vi "Measurement Data Convert (Harmonics).vi"(7 "Number of Harmonics Order (1)":i32=1 min=1 max=32, 8 "error in (no error)":errorcluster, 9 "Item Number Offset (1)":i32=1 min=1 max=32, 10 "Measurement Data (Empty)":string, 11 "VISA resource name":refnum<visa-resource-name>) -> (0 "error out":errorcluster, 1 "Measurement":dbl[][](array[numeric]), 2 "Function":string[](array[string]), 3 "VISA resource name out":refnum<visa-resource-name>)   [LabVIEW 2023, in "Yokogawa WT300 Series.lvlib"]
doc: "Transforms measurement datas into harmonics numeric data list values."
uses:
  Yokogawa WT300 Series.lvlib
panel:
  # "Total        DC            1             2              3             4"
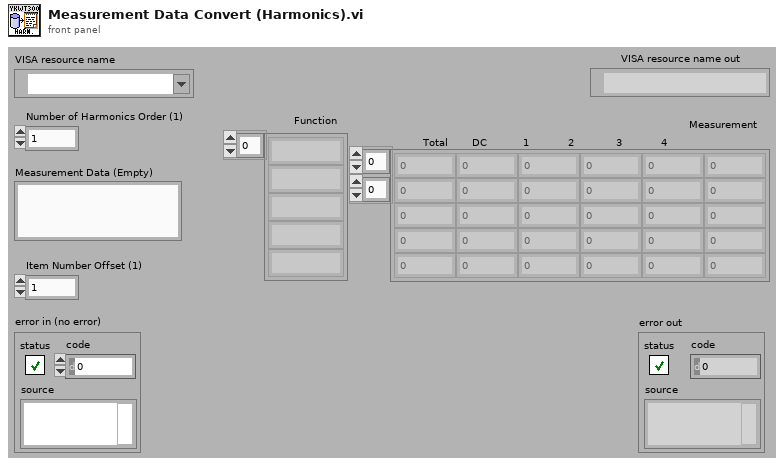
[diagram p1: front panel]
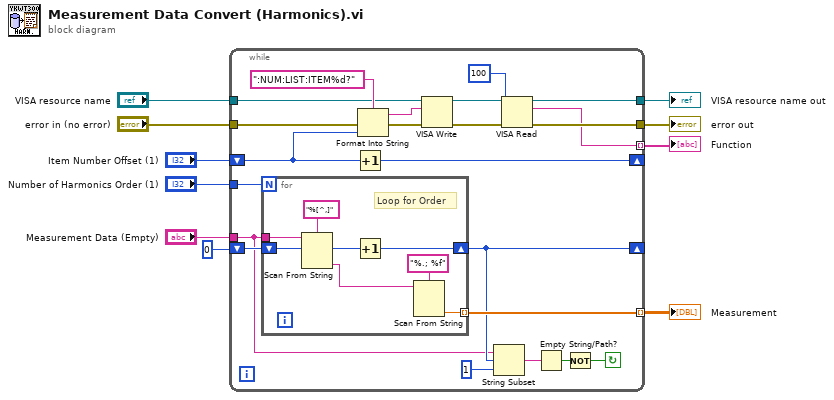
[diagram p0: block diagram]
diagram:
  n1 = while {
    tunnel: [w31] -> w4 mode=indexing
    tunnel: "Measurement Data (Empty)" -> [w23]
    shift-right: [w24] -> _
    shift-left: 0 -> [w32]
    tunnel: "VISA resource name" -> [w20]
    tunnel: "error in (no error)" -> [w22]
    shift-right: [w30] -> _
    shift-left: "Item Number Offset (1)" -> [w17]
    tunnel: [w13] -> w7
    tunnel: [w12] -> w6
    tunnel: [w11] -> w5 mode=indexing
    tunnel: "Number of Harmonics Order (1)" -> [w29]
    stop <- w25 continue-if-true
    n2 = for {
      N: w29 -> [_]
      tunnel: w23 -> [w33]
      tunnel: [w36] -> w31 mode=indexing
      shift-right: [w34] -> w24
      shift-left: w32 -> [w39]
      # "Loop for Order"
      n3 = Scan From String(format string="%[^,]", input string=w33, initial scan location=w39) -> (offset past scan=w38:u32, output 1=w37:string)  [unwired: 2 in, 2 out]
      n4 = Increment(x=w38) -> (x+1=w34:u32)
      n5 = Scan From String(format string="%.; %f" ("形式文字列"), input string=w37) -> (output 1=w36:dbl)  [unwired: 3 in, 3 out]
    }
    n6 = Increment(x=w17) -> (x+1=w30:i32)
    n7 = Format Into String(format string=":NUM:LIST:ITEM%d?" ("形式文字列"), error in=w22, w17) -> (resulting string=w19:string, error out=w18:errorcluster)  [unwired: 1 in]
    n8 = VISA Write ("VISA書き込み")(VISA resource name=w20, write buffer=w19, error in (no error)=w18) -> (VISA resource name out=w15:refnum<visa-resource-name>, error out=w14:errorcluster)  [unwired: 1 out]
    n9 = String Subset(string=w23, offset (0)=w24, length (rest)=1) -> (substring=w27:string)
    n10 = VISA Read ("VISA読み取り")(VISA resource name=w15, byte count=u32 100, error in (no error)=w14) -> (VISA resource name out=w13:refnum<visa-resource-name>, read buffer=w11:string, error out=w12:errorcluster)  [unwired: 1 out]
    n11 = Empty String/Path?(string/path=w27) -> (empty?=w28:bool)
    n12 = Not(x=w28) -> (.not. x?=w25:bool)
  }
  "error out" <- w6
  "VISA resource name out" <- w7
  "Measurement" <- w4
  "Function" <- w5
